vi "Pre Launch Init.vi"(11 "Nested in":refnum<class "Serial Devices.lvclass">) -> (0 "error out":errorcluster, 3 "Nested out":refnum<class "Serial Devices.lvclass">)   [LabVIEW 2019, in "Serial Devices.lvlib" / "Serial Devices.lvclass"]
doc: "(<B>Filename</B>: Actor Framework.lvlib:Actor.lvclass:Pre Launch Init.vi)\n\nDefines behavior that occurs after the Launch Nested Actor method is invoked but before the actor's Actor Core method begins running.\n\nBy default, this method does nothing. A descendant class may override it to define behavior."
uses:
  Serial Devices.lvclass
  C:/Program Files (x86)/National Instruments/LabVIEW 2019/vi.lib/ActorFramework/Actor/Actor.lvclass
  Serial Devices.lvclass/Serial Devices.ctl
  <vilib>/ActorFramework/Actor/Actor.lvclass/Actor.ctl
  <vilib>/ActorFramework/Message Enqueuer/Message Enqueuer.lvclass/Message Enqueuer.ctl
  <vilib>/ActorFramework/Message Enqueuer/Init from Existing Queue.vi
  <vilib>/ActorFramework/Message Enqueuer/Enqueue.vi
  Serial Devices Messages/Init Msg/Init Msg.lvclass
  C:/Program Files (x86)/National Instruments/LabVIEW 2019/vi.lib/ActorFramework/Message/Message.lvclass
  Serial Devices Messages/Crear Conexion Msg/Crear Conexion Msg.lvclass
  <vilib>/ActorFramework/Message Priority Queue/Priority Enqueue.vi
  <vilib>/ActorFramework/Message Enqueuer/Message Enqueuer.lvclass
  <vilib>/ActorFramework/Actor/Actor.lvclass
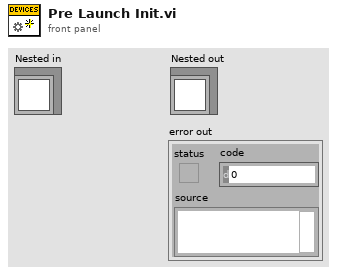
[diagram p1: front panel]
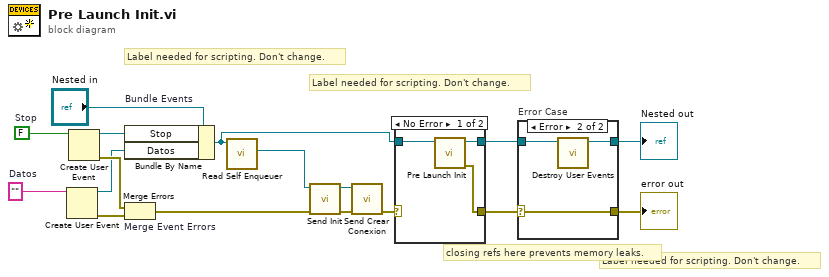
[diagram p0: block diagram]
diagram:
  w3 = ""  # Datos
  w16 = FALSE  # Stop
  # "Label needed for scripting. Don't change."
  # "Label needed for scripting. Don't change."
  # "Label needed for scripting. Don't change."
  # "closing refs here prevents memory leaks."
  n1 = Create User Event(user event datatype=w3) -> (user event=w2:refnum<user-event>, error out=w1:errorcluster)  [unwired: 1 in]
  n2 = Create User Event(user event datatype=w16) -> (user event=w13:refnum<user-event>, error out=w15:errorcluster)  [unwired: 1 in]
  n3 = Bundle By Name "Bundle Events"(cluster="Nested in", "Stop"=w13, "Datos"=w2) -> (w9:refnum<class "Serial Devices.lvclass">)
  n4 = Merge Errors "Merge Event Errors"(w15, w1) -> (w7:errorcluster)
  n5 = call <vilib>:"Read Self Enqueuer.vi"("Actor"=w9) -> ("Self Enqueuer"=w8:refnum<class "Message Enqueuer.lvclass">)  [unwired: 10 in]
  n6 = call "Send Init.vi"("error in (no error)"=w7, "Message Enqueuer"=w8) -> ("error out"=w5:errorcluster, "Message Enqueuer out"=w6:refnum<class "Message Enqueuer.lvclass">)  [unwired: 8 in]
  n7 = call "Send Crear Conexion.vi"("error in (no error)"=w5, "Message Enqueuer"=w6) -> ("error out"=w4:errorcluster)  [unwired: 8 in, 1 out]
  n8 = case shown="No Error" w4 {
    selector: w4 -> [_ w22]
    tunnel: [w20 w21] -> w11
    tunnel: w9 -> [w19 w21]
    tunnel: [w18 w22] -> w10
    frame No Error {
      n9 = call-parent "Pre Launch Init.vi"("Actor in"=w19) -> ("error out"=w18:errorcluster, "Actor out"=w20:refnum<class "Serial Devices.lvclass">)  [unwired: 9 in]
    }
    frame Error {
    }
  }
  n10 = case "Error Case" shown="Error" w10 {
    selector: w10 -> [w23 w27]
    tunnel: w11 -> [w24 w26]
    tunnel: [w24 w25] -> w14
    tunnel: [w23 w27] -> w12
    frame No Error {
    }
    frame Error {
      n11 = call "Destroy User Events.vi"("UI Template in"=w26) -> ("UI Template out"=w25:refnum<class "Serial Devices.lvclass">)  [unwired: 10 in]
    }
  }
  "error out" <- w12
  "Nested out" <- w14
